vi "Get Alternative List Value.vi"(2 "Current Value":string, 3 "List in":string[](array[string])) -> (0 "Altenative Value":string, 1 "Alternative Available":bool)   [LabVIEW 2020, in "Test.Camera.lvclass"]
uses:
  Test.Camera.lvclass
  Test.Camera.lvclass/Test.Camera.ctl
  1a5b698b-b1e6-4ec2-a46b-3d59f4d11909.vi
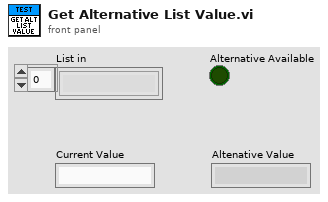
[diagram p1: front panel]
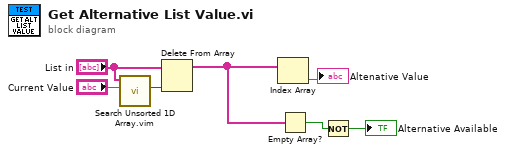
[diagram p0: block diagram]
diagram:
  n1 = call "Search Unsorted 1D Array.vim"("element"="Current Value", "unsorted 1D array"="List in") -> ("index of element"=w6:i32)  [unwired: 9 in]
  n2 = Delete From Array(array="List in", index=w6) -> (array with subset deleted=w3:string[])  [unwired: 1 in, 1 out]
  n3 = Index Array(array=w3) -> (element=→"Altenative Value":string)  [unwired: 1 in]
  n4 = Empty Array?(array=w3) -> (empty?=w2:bool)
  n5 = Not(x=w2) -> (.not. x?=→"Alternative Available":bool)
